vi "test AE - Radial Graph Data.vi"() -> ()   [LabVIEW 2017]
doc: "Developed by Kevin Thompson\nkevin@thompsonengineering.net\n\nCopyright 2018-2020\nThompson Engineering, LLC"
uses:
  LV_Source/Application/DataTypes/TD Action - AE - Radial Graph manager --enum.ctl
  <userlib>/_OpenG.lib/numeric/numeric.llb/Random Number Within Range - DBL__ogtk.vi
  LV_Source/Application/Application.lvclass
panel:
  out "error out":errorcluster
  in  "stop":bool
  out "Scaled Vfb":dbl
  out "Vsp SF":dbl
  out "XY Graph":cluster{dbl[], dbl[]}[](graph)=[{[9.998476951563912], [-0.1745240643728356]}, {array[360 elements], array[360 elements]}, {array[360 elements], array[360 elements]}, {array[360 elements], array[360 elements]}]
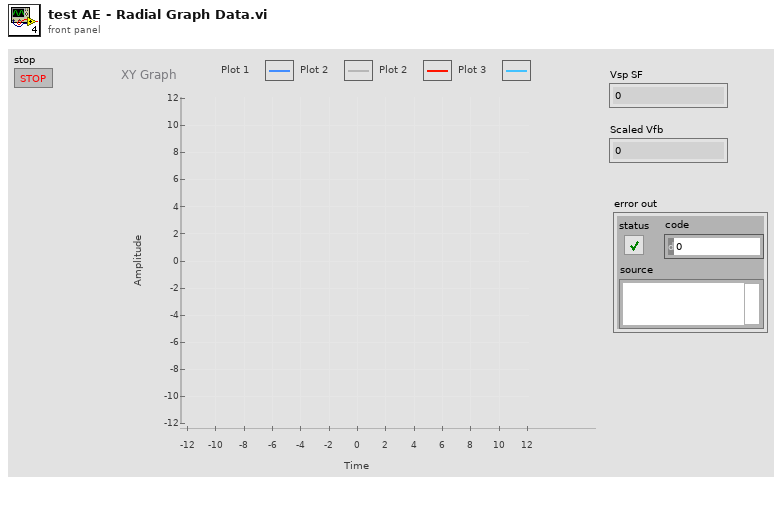
[diagram p1: front panel]
types:
  T1 = typedef "Application.lvclass/TD Action - AE - Radial Graph manager --enum.ctl" = enum16{"NoOp", "Init_AE", "Init GraphData", "Input Data", "Input TTPos Only", "Clear V-FB"}
  T2 = typedef "CartesianForm_RadialGraphData_AllPlots--cluster.ctl" = cluster{"TT Pos":T3, "TT Circle":T3, "V-FB":T3, "V-SP":T3}
  T3 = typedef "CartesianForm_GraphPlotData--cluster.ctl" = cluster{"X[]":dbl[], "Y[]":dbl[]}
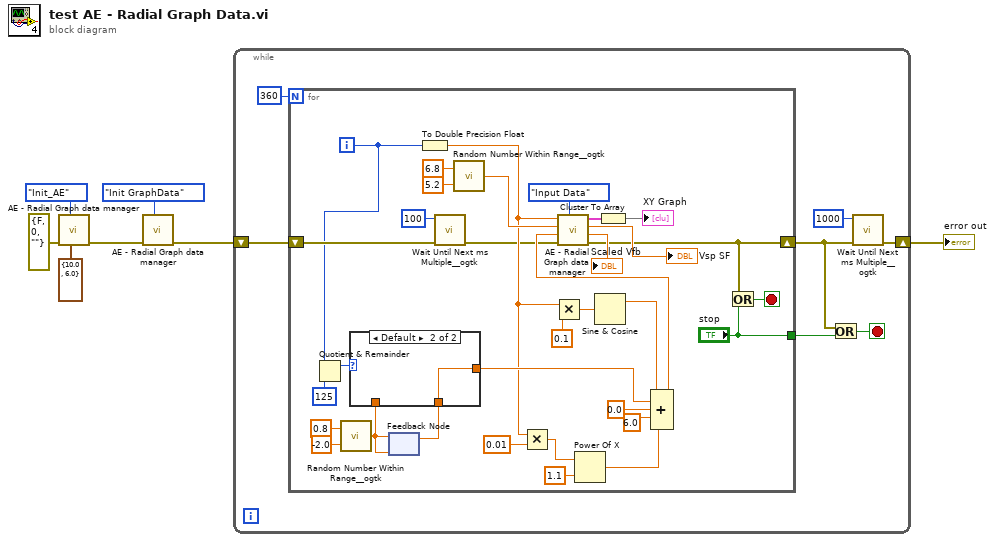
[diagram p0: block diagram]
diagram:
  n1 = call "AE - Radial Graph data manager.vi"("Nominal Radius"=cluster{"outer ring":dbl, "inner ring":dbl} {"outer ring"=10.0, "inner ring"=6.0}, "Action (NoOp)"=TD_Action_-_AE_-_Radial_Graph_manager_--enum."Init_AE", "error in (no error)"=errorcluster {"status"=FALSE, "code"=0, "source"=""}) -> ("error out"=w5:errorcluster)  [unwired: 5 in, 3 out]
  n2 = call "AE - Radial Graph data manager.vi"("Action (NoOp)"=TD_Action_-_AE_-_Radial_Graph_manager_--enum."Init GraphData", "error in (no error)"=w5) -> ("error out"=w4:errorcluster)  [unwired: 6 in, 3 out]
  n3 = while {
    shift-right: [w10] -> w3
    shift-left: w4 -> [w14]
    stop <- w12 stop-if-true
    n4 = for {
      N: 360 -> [_]
      shift-right: [w16] -> w11
      shift-left: w14 -> [w46]
      tunnel: ["stop"] -> w8
      i -> [w24]
      stop <- w17 stop-if-true
      n5 = Quotient & Remainder(x=w24, y=125) -> (x-y*floor(x/y)=w32:i32)  [unwired: 1 out]
      n6 = call-poly <userlib>:"Random Number Within Range__ogtk.vi"("High"=0.8, "Low"=-2.0) -> ("Random Number"=w28:dbl)  [unwired: 3 in]
      n7 = feedback #1(w28) -> (w27:dbl)
      n8 = case shown="Default" w32 {
        tunnel: w28 -> [w48 _]
        tunnel: w27 -> [_ w49]
        tunnel: [w48 w49] -> w25
        frame 0 {
        }
        frame Default {
        }
      }
      n9 = feedback-in #1(w28) -> ()
      n10 = To Double Precision Float(number=w24) -> (double precision float=w23:dbl)
      n11 = call <userlib>:"Wait Until Next ms Multiple__ogtk.vi"("error in (no error)"=w46, "milliseconds to wait"=u32 100) -> ("error out"=w19:errorcluster)  [unwired: 8 in, 1 out]
      n12 = call-poly <userlib>:"Random Number Within Range__ogtk.vi"("High"=6.8, "Low"=5.2) -> ("Random Number"=w43:dbl)  [unwired: 3 in]
      n13 = Multiply(x=w23, y=0.01) -> (x*y=w34:dbl)
      n14 = Multiply(x=w23, y=0.1) -> (x*y=w40:dbl)
      n15 = Power Of X(1:1.1 ("x"), 2:w34) -> (0:w33:dbl)
      n16 = Sine & Cosine(0:w40) -> (1:w26:dbl)  [unwired: 1 out]
      n17 = Compound Arithmetic op=ADD(w26, w25, 0.0 ("value"), 6.0 ("circle radius"), w33) -> (w22:dbl)
      n18 = call "AE - Radial Graph data manager.vi"("Action (NoOp)"=TD_Action_-_AE_-_Radial_Graph_manager_--enum."Input Data", "error in (no error)"=w19, "Vfb"=w22, "VspSum"=w43, "TTPos (deg)"=w23) -> ("error out"=w16:errorcluster, "Scaled Vfb"=→"Scaled Vfb":dbl, "Vsp SF"=→"Vsp SF":dbl, "RadialGraphAllPlotsData"=w45:T2)  [unwired: 3 in]
      n19 = Cluster To Array(cluster=w45) -> (array=→"XY Graph":T3[])
      n20 = Or(x=w16, y="stop") -> (x .or. y?=w17:bool)
    }
    n21 = Or(x=w11, y=w8) -> (x .or. y?=w12:bool)
    n22 = call <userlib>:"Wait Until Next ms Multiple__ogtk.vi"("error in (no error)"=w11, "milliseconds to wait"=u32 1000) -> ("error out"=w10:errorcluster)  [unwired: 8 in, 1 out]
  }
  "error out" <- w3
